vi "PithegoreanTheorem.vi"(8 "b":dbl, 11 "a":dbl) -> (1 "c":dbl)   [LabVIEW 2014]
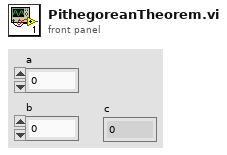
[diagram p1: front panel]
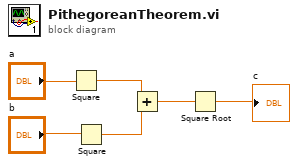
[diagram p0: block diagram]
diagram:
  n1 = Square(x="a") -> (x^2=w4:dbl)
  n2 = Square(x="b") -> (x^2=w3:dbl)
  n3 = Add(x=w4, y=w3) -> (x+y=w2:dbl)
  n4 = Square Root(x=w2) -> (sqrt(x)=→"c":dbl)
